vi "Size.vi"(8 "error in (no error)":errorcluster, 11 "Path Array in":refnum<class "Path Array.lvclass">) -> (0 "error out":errorcluster, 2 "Size":i32, 3 "Path Array out":refnum<class "Path Array.lvclass">)   [LabVIEW 2020, in "Data.lvlib" / "Path Array.lvclass"]
doc: "Return the size of the generic data element."
uses:
  Path Array.lvclass
  Path Array.lvclass/Path Array.ctl
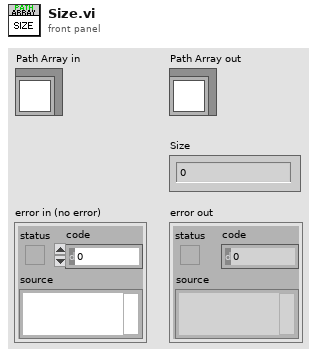
[diagram p1: front panel]
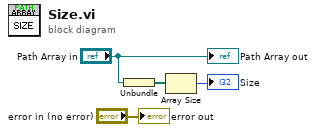
[diagram p0: block diagram]
diagram:
  n1 = Unbundle("Path Array in") -> (w2:path[])
  n2 = Array Size(array=w2) -> (size(s)=→"Size":i32)
  "error out" <- "error in (no error)"
  "Path Array out" <- "Path Array in"
